vi "ep_Configure Settings.vi"(0 "spectra settings":T5={"number of lines"=12501, "% overlap"=0.0, "maximum frequency [Hz]"=250.0}, 5 "parameters":T2, 11 "error in (no error)":errorcluster) -> (4 "initial conditions":T3 {"zoom FFT settings"."FFT settings"."window" items=["Rectangle"=0, "Hanning"=1, "Hamming"=2, "Blackman-Harris"=3, "Exact Blackman"=4, "Blackman"=5, "Flat Top"=6, "4 Term B-Harris "=7, "7 Term B-Harris"=8, "Low Sidelobe"=9, "Blackman Nuttall"=11, "Triangle"=30, "Bartlett-Hanning"=31, "Bohman"=32, "Parzen"=33, "Welch"=34, "Kaiser"=60, "Dolph-Chebyshev"=61, "Gaussian"=62]}, 15 "error out":errorcluster)   [LabVIEW 2014, in "NI_EP_Motor Monitoring.lvlib"]
uses:
  <vilib>/addons/Electrical Power/Motor Monitoring/NI_EP_Motor Monitoring.lvlib
  <vilib>/addons/Electrical Power/Motor Monitoring/subVIs/ep_Spectra Settings.ctl
  <vilib>/addons/Electrical Power/Motor Monitoring/subVIs/ep_Initial Conditions for MCSA Spectra.ctl
  <vilib>/addons/Electrical Power/Motor Monitoring/subVIs/ep_Demodulation Algorithm.ctl
  <vilib>/addons/Electrical Power/Motor Monitoring/subVIs/ep_Zoom FFT Settings.ctl
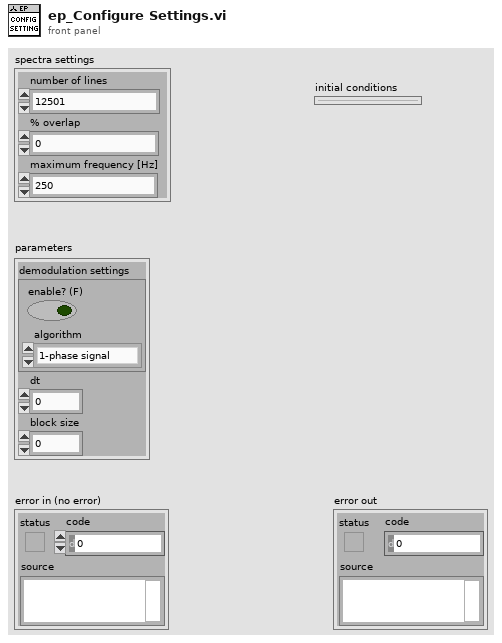
[diagram p1: front panel]
types:
  T1 = typedef "NI_EP_Motor Monitoring.lvlib/ep_Demodulation Algorithm.ctl" = enum16{"1-phase signal", "3-phase signals"}
  T2 = cluster{"demodulation settings":cluster{"enable? (F)":bool, "algorithm":T1}, "dt":dbl, "block size":i32}
  T3 = typedef "NI_EP_Motor Monitoring.lvlib/ep_Initial Conditions for MCSA Spectra.ctl" = cluster{"hilbert state":cluster{"delay conditions":dbl[], "filter conditions":dbl[]}, "zoom FFT state":cluster{"phase state":dbl, "zoom FFT state":cluster{"zoom settings state":cluster{"zoom":i32, "stop band attenuation":enum16{"84 dB", "96 dB", "120 dB"}, "alias protect in final transition":bool, "oversampling ratio":dbl}, "SML Decimation Filter (complex input) state":cluster{"decimation settings state":cluster{"M":i32, "stop band attenuation":enum16{"84 dB", "96 dB", "120 dB"}, "alias protect in transition band":bool, "oversampling ratio":dbl}, "counter for garbage samples state":i32, "sml_Parameter Setting for Zoom Factor state":cluster{"filter length * interpolation state":i32, "interpolation state":i32, "comb filter order state":i32, "CFIR par state":cluster{"h":dbl[], "M":i32, "N":i32}, "LFIR par state":cluster{"h":dbl[], "M":i32, "N":i32}, "CIC Stages state":i32}, "aal_CIC (complex input) state":cluster{"aal_cascaded moving average (complex input) state":cluster{"states":cdb[], "circular buffers state":cdb[][], "circular buffer counter state":i32}, "aal_moving average with decimation by order (complex input) state":cluster{"residue result state":cdb, "processed data counter state":i32}}, "sml_Cascaded Decimation Filter (complex input) CFIR state":cluster{"unprocessed data state":cdb[], "final conditions state":cdb[][], "sml_M-1 Decimator with IC (complex input) state":cluster{"coefficients in reverse order state":dbl[], "max index for coefficients state":i32}}, "sml_Cascaded Decimation Filter (complex input) LFIR state":cluster{"unprocessed data state":cdb[], "final conditions state":cdb[][], "sml_M-1 Decimator with IC (complex input) state":cluster{"coefficients in reverse order state":dbl[], "max index for coefficients state":i32}}}, "ma_SML Data Packing (complex input) state":cluster{"array getting packed state":cdb[], "last array processed state":cdb[], "index state":i32, "packing parameters state":cluster{i32, "size":i32}}}, "FFT{X} [Vrms]":cdb[]}, "IIR filter state":cluster{"filter state":dbl[]}, "demodulation settings":cluster{"enable? (F)":bool, "algorithm":T1}, "highpass IIR Filter":cluster{"filter structure":enum32{"IIR 2nd Order", "IIR 4th Order"}, "Reverse Coefficients":dbl[], "Forward Coefficients":dbl[]}, "Hilbert FIR filter":cluster{"coefficients":dbl[], "delay":i32}, "zoom FFT settings":T4}
  T4 = typedef "NI_EP_Motor Monitoring.lvlib/ep_Zoom FFT Settings.ctl" = cluster{"FFT settings":cluster{"window":u16, "Window Size":i32, "FFT Size":i32, "%overlap":dbl}, "zoom settings":cluster{"zoom":i32, "stop band attenuation":enum16{"84 dB", "96 dB", "120 dB"}, "alias protect in final transition":bool, "oversampling ratio":dbl}, "other settings":cluster{"fmod":dbl, "f0":dbl, "df":dbl, "oidx":i32, "olen":i32}, "iterations":i32, "max block size":i32, "fs":dbl}
  T5 = typedef "NI_EP_Motor Monitoring.lvlib/ep_Spectra Settings.ctl" = cluster{"number of lines":i32, "% overlap":dbl, "maximum frequency [Hz]":dbl}
  T6 = cluster{"filter structure":enum32{"IIR 2nd Order", "IIR 4th Order"}, "Reverse Coefficients":dbl[], "Forward Coefficients":dbl[]}
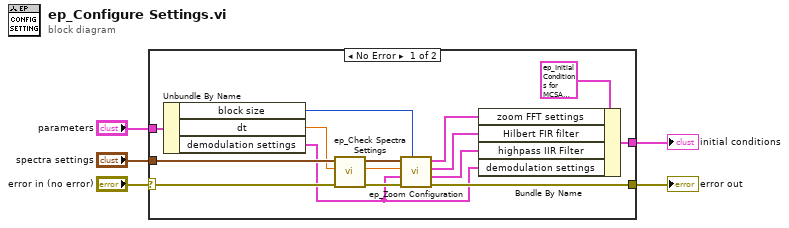
[diagram p0: block diagram]
diagram:
  n1 = case shown="No Error" "error in (no error)" {
    selector: "error in (no error)" -> [w17 w21]
    tunnel: [w16 w21] -> w4
    tunnel: "spectra settings" -> [w15 _]
    tunnel: [w11 _] -> w1
    tunnel: "parameters" -> [w10 _]
    frame No Error {
      n2 = Unbundle By Name(w10) -> ("block size"=w8:i32, "dt"=w7:dbl, "demodulation settings"=w9:cluster{"enable? (F)":bool, "algorithm":T1})
      n3 = call <vilib>:"ep_Check Spectra Settings.vi"("error in (no error)"=w17, "dt"=w7, "spectra settings"=w15) -> ("error out"=w18:errorcluster, "fs"=w19:dbl, "dup spectra settings"=w20:T5)  [unwired: 6 in]
      n4 = call <vilib>:"ep_Zoom Configuration.vi"("block size"=w8, "error in (no error)"=w18, "demodulation settings"=w9, "fs"=w19, "spectra settings"=w20) -> ("error out"=w16:errorcluster, "highpass IIR Filter"=w14:T6, "Hilbert FIR filter"=w12:cluster{"coefficients":dbl[], "delay":i32}, "zoom FFT settings"=w13:T4)  [unwired: 3 in]
      n5 = Bundle By Name(cluster=T3 {"hilbert state"={"delay conditions"=[], "filter conditions"=[]}, "zoom FFT state"={"phase state"=0.0, "zoom FFT state"={"zoom settings state"={"zoom"=0, "stop band attenuation"=enum."84 dB", "alias protect in final transition"=FALSE, "oversampling ratio"=0.0}, "SML Decimation Filter (complex input) state"={"decimation settings state"={"M"=0, "stop band attenuation"=enum."84 dB", "alias protect in transition band"=FALSE, "oversampling ratio"=0.0}, "counter for garbage samples state"=0, "sml_Parameter Setting for Zoom Factor state"={"filter length * interpolation state"=0, "interpolation state"=0, "comb filter order state"=0, "CFIR par state"={"h"=[], "M"=0, "N"=0}, "LFIR par state"={"h"=[], "M"=0, "N"=0}, "CIC Stages state"=0}, "aal_CIC (complex input) state"={"aal_cascaded moving average (complex input) state"={"states"=[], "circular buffers state"=[], "circular buffer counter state"=0}, "aal_moving average with decimation by order (complex input) state"={"residue result state"=0.0+0.0i, "processed data counter state"=0}}, "sml_Cascaded Decimation Filter (complex input) CFIR state"={"unprocessed data state"=[], "final conditions state"=[], "sml_M-1 Decimator with IC (complex input) state"={"coefficients in reverse order state"=[], "max index for coefficients state"=0}}, "sml_Cascaded Decimation Filter (complex input) LFIR state"={"unprocessed data state"=[], "final conditions state"=[], "sml_M-1 Decimator with IC (complex input) state"={"coefficients in reverse order state"=[], "max index for coefficients state"=0}}}, "ma_SML Data Packing (complex input) state"={"array getting packed state"=[], "last array processed state"=[], "index state"=0, "packing parameters state"={0, "size"=0}}}, "FFT{X} [Vrms]"=[]}, "IIR filter state"={"filter state"=[]}, "demodulation settings"={"enable? (F)"=FALSE, "algorithm"=enum."1-phase signal"}, "highpass IIR Filter"={"filter structure"=enum."IIR 2nd Order", "Reverse Coefficients"=[], "Forward Coefficients"=[]}, "Hilbert FIR filter"={"coefficients"=[], "delay"=0}, "zoom FFT settings"={"FFT settings"={"window"=0, "Window Size"=0, "FFT Size"=0, "%overlap"=0.0}, "zoom settings"={"zoom"=0, "stop band attenuation"=enum."84 dB", "alias protect in final transition"=FALSE, "oversampling ratio"=0.0}, "other settings"={"fmod"=0.0, "f0"=0.0, "df"=0.0, "oidx"=0, "olen"=0}, "iterations"=0, "max block size"=0, "fs"=0.0}} ("initial conditions"), "zoom FFT settings"=w13, "Hilbert FIR filter"=w12, "highpass IIR Filter"=w14, "demodulation settings"=w9) -> (w11:T3)
    }
    frame Error {
    }
  }
  "error out" <- w4
  "initial conditions" <- w1
